vi "TL create normal distribution.vi"(1 "std (Normal)":dbl=5.0 format="%#_13g", 2 "mean":dbl) -> (0 "ACT array":dbl[](array[numeric]))   [LabVIEW 2014]
doc: "This VI creates an array to be used by the midbrain arbiter. It calulates a normal distribution based upon the passed mean with an std of 5."
uses:
  <vilib>/Analysis/1siggen.llb/Ramp Pattern by Samples.vi
  <vilib>/gmath/statdist.llb/Normal PDF.vi
  <vilib>/gmath/NI_Gmath.lvlib
  <vilib>/Analysis/NI_AALBase.lvlib
panel:
  out "ACT array Graph":cluster{dbl, dbl, dbl[]}(graph)
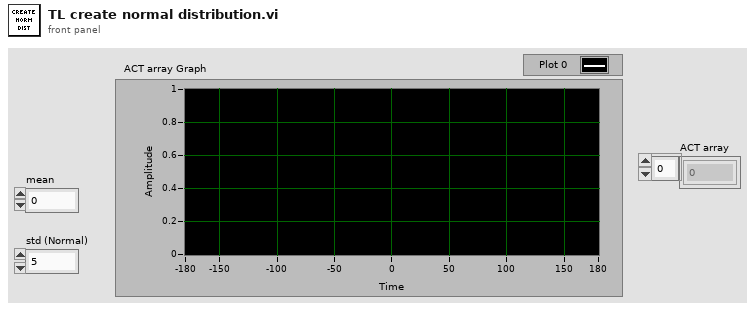
[diagram p1: front panel]
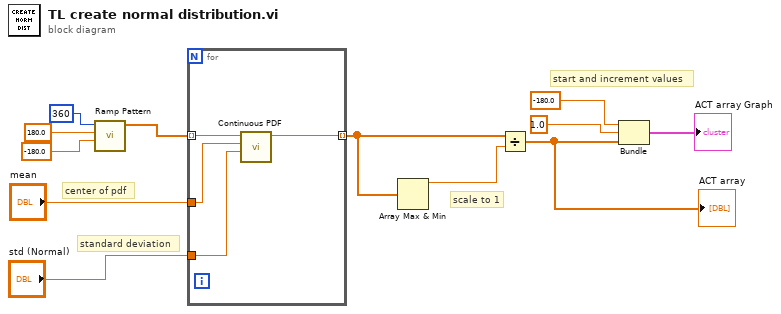
[diagram p0: block diagram]
diagram:
  # "standard deviation"
  # "center of pdf"
  # "start and increment values"
  # "scale to 1"
  n1 = call-poly <vilib>:"Ramp Pattern.vi"("start"=-180.0, "end"=180.0, "samples"=360) -> ("Ramp Pattern"=w10:dbl[])  [unwired: 7 in, 1 out]
  n2 = for {
    tunnel: w10 -> [w13] mode=indexing
    tunnel: "std (Normal)" -> [w16]
    tunnel: [w15] -> w4 mode=indexing
    tunnel: "mean" -> [w14]
    n3 = call-poly <vilib>:"Continuous PDF.vi"("std"=w16, "mean"=w14, "x"=w13) -> ("pdf(x)"=w15:dbl)  [unwired: 7 in, 1 out]
  }
  n4 = Array Max & Min(array=w4) -> (max value=w3:dbl)  [unwired: 3 out]
  n5 = Divide(x=w4, y=w3) -> (x/y=w2:dbl[])
  "ACT array" <- w2
  n6 = Bundle(-180.0, 1.0, w2) -> (→"ACT array Graph":cluster{dbl, dbl, dbl[]})  [unwired: 1 in]
